vi "Write_Document.vi"(8 "error in (no error)":errorcluster caption="entrée d'erreur (pas d'erreur)", 10 "Input.Document":string, 11 "Firebase (Default) en entrée":refnum<class "Firebase Driver.lvclass">) -> (0 "error out":errorcluster caption="sortie d'erreur", 3 "Firebase (Default) en sortie":refnum<class "Firebase Driver.lvclass">)   [LabVIEW 2020, in "Library Instrument & Equipement.lvlib" / "Library FireBase.lvlib" / "Firebase Driver.lvclass"]
uses:
  Firebase Driver.lvclass
  Firebase Driver.lvclass/Firebase Driver.ctl
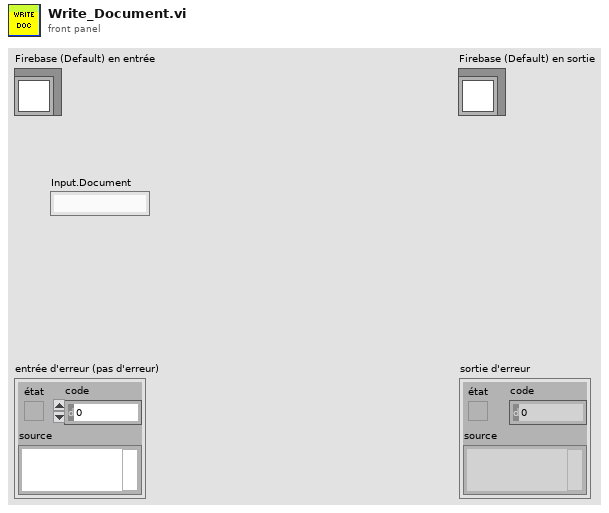
[diagram p1: front panel]
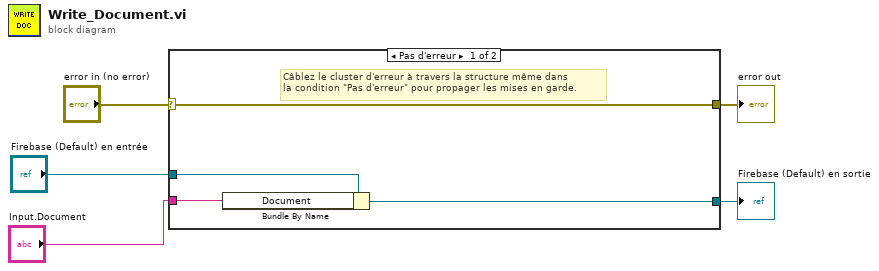
[diagram p0: block diagram]
diagram:
  n1 = case shown="Pas d'erreur" "error in (no error)" {
    selector: "error in (no error)" -> [w9 w11]
    tunnel: [w9 w11] -> w4
    tunnel: [w7 w10] -> w2
    tunnel: "Firebase (Default) en entrée" -> [w8 w10]
    tunnel: "Input.Document" -> [w6 _]
    frame No Error {
      # "Câblez le cluster d'erreur à travers la structure même dans\nla condition \"Pas d'erreur\" pour propager les mises en garde."
      n2 = Bundle By Name(cluster=w8, "Document"=w6) -> (w7:refnum<class "Firebase Driver.lvclass">)
    }
    frame Error {
    }
  }
  "error out" <- w4
  "Firebase (Default) en sortie" <- w2
